vi "DigitalOutTriggerSet.vi"(8 "error in (no error)":errorcluster caption="错误输入（无错误）", 9 "trigcond":enum16{"Raising", "Falling", "Either"}(ring), 10 "trigsrc":T1(ring), 11 "handle":u64) -> (0 "error out":errorcluster caption="错误输出", 2 "function return":i32, 3 "handle out":u64)   [LabVIEW 2018]
doc: "Set pos. or neg. Supply voltage"
uses:
  InstrumentsPlayground.lvlib
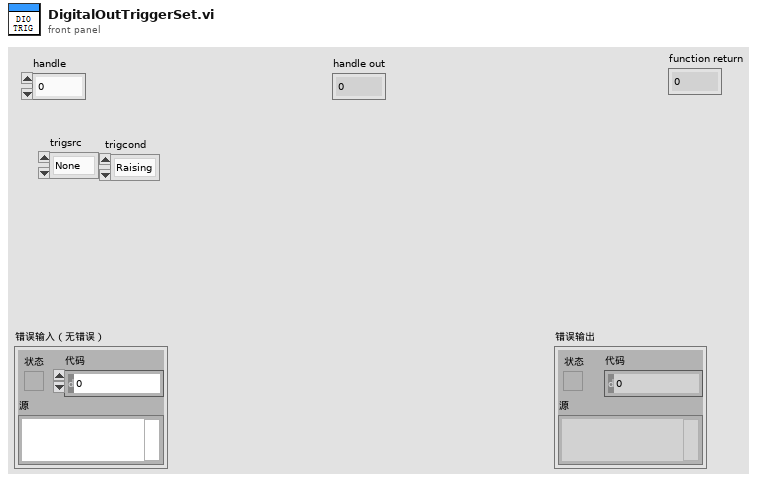
[diagram p1: front panel]
types:
  T1 = enum16{"None", "DetectorAnalogInCH1", "DetectorAnalogInCH2", "AnalogOut1", "AnalogOut2", "DetectorDigitalIn", "DigitalOut", "Manule", "External 1", "External 2", "DigitalIn"}
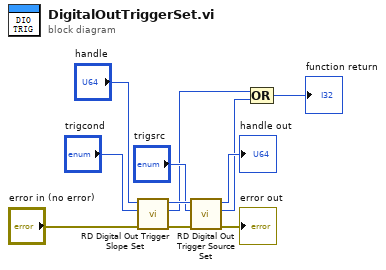
[diagram p0: block diagram]
diagram:
  n1 = call "RD Digital Out Trigger Slope Set.vi"("error in (no error)"="error in (no error)", "slope"="trigcond", "handle"="handle") -> ("error out"=w10:errorcluster, "function return"=w1:i32, "handle out"=w8:u64)  [unwired: 6 in]
  n2 = call "RD Digital Out Trigger Source Set.vi"("error in (no error)"=w10, "trigsrc"="trigsrc", "handle"=w8) -> ("error out"=→"error out":errorcluster, "function return"=w3:i32, "handle out"=→"handle out":u64)  [unwired: 6 in]
  n3 = Compound Arithmetic op=OR(w1, w3) -> (→"function return":i32)
